vi "RunCore.vi"(8 "ErrorIn":errorcluster, 9 "Timeout (s)":dbl, 10 "MeasIn":refnum<class "VoltageMeas.lvclass">, 11 "RefIn":refnum<class "IReference.lvclass">) -> (0 "ErrorOut":errorcluster, 1 "Timeout?":bool, 2 "ResultOut":refnum<class "IResult.lvclass">, 3 "RefOut":refnum<class "IReference.lvclass">)   [LabVIEW 2019, in "VoltageMeas.lvclass"]
uses:
  VoltageMeas.lvclass
  DMM/DMM.lvclass
  VoltageResult/VoltageResult.lvclass
  C:/Repo/LabVIEW-SOLID-Examples/Architecture/IReference/IReference.lvclass
  C:/Repo/LabVIEW-SOLID-Examples/Architecture/IResult/IResult.lvclass
  IReference/IReference.lvclass
  IResult/IResult.lvclass
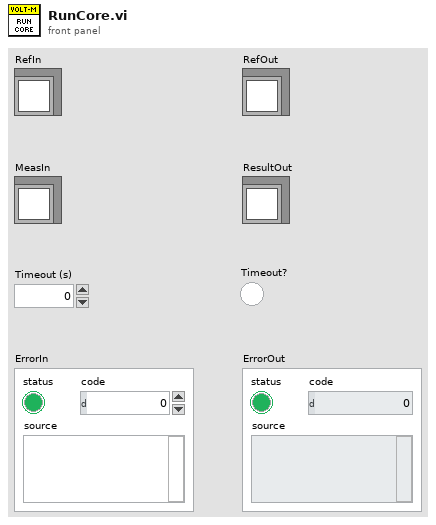
[diagram p1: front panel]
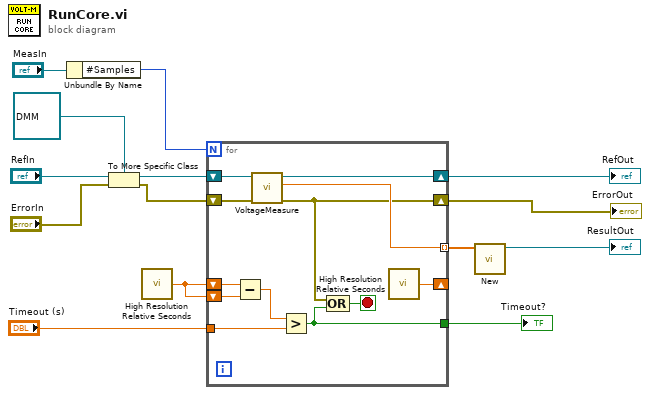
[diagram p0: block diagram]
diagram:
  n1 = Unbundle By Name("MeasIn") -> ("#Samples"=w8:i32)
  n2 = To More Specific Class(target class=refnum<class "DMM.lvclass"> refnum ("DMM.lvclass"), reference="RefIn", error in="ErrorIn") -> (specific class reference=w12:refnum<class "DMM.lvclass">, error out=w10:errorcluster)
  n3 = call <vilib>:"High Resolution Relative Seconds.vi"() -> ("relative seconds"=w4:dbl)
  n4 = for {
    N: w8 -> [_]
    shift-right: [w17] -> w1
    shift-left: w10 -> [w25]
    shift-right: [w24] -> w7
    shift-left: w12 -> [w26]
    tunnel: [w23] -> w6 mode=indexing
    shift-right: [w18] -> _
    shift-left: w4 -> [w22]
    shift-left: w4 -> [w21]
    tunnel: "Timeout (s)" -> [w19]
    tunnel: [w15] -> w2
    stop <- w16 stop-if-true
    n5 = Subtract(x=w22, y=w21) -> (x-y=w20:dbl)
    n6 = call "VoltageMeasure.vi"("Error In"=w25, "DMMIn"=w26) -> ("Error Out"=w17:errorcluster, "Measurement"=w23:dbl, "DMMOut"=w24:refnum<class "DMM.lvclass">)  [unwired: 7 in]
    n7 = Greater?(x=w20, y=w19) -> (0:w15:bool)
    n8 = Compound Arithmetic op=OR(w17, w15) -> (w16:bool)
    n9 = call <vilib>:"High Resolution Relative Seconds.vi"() -> ("relative seconds"=w18:dbl)
  }
  "ErrorOut" <- w1
  "RefOut" <- w7
  "Timeout?" <- w2
  n10 = call "New.vi"("VoltageMeasArray"=w6) -> ("VoltageResult.lvclass"=→"ResultOut":refnum<class "VoltageResult.lvclass">)  [unwired: 10 in]
